vi "Set Parameters File MD5 Checksum.vi"(8 "error in":errorcluster, 9 "MD5":string, 11 "custom device ref":T1 format="%.0x") -> (0 "error out":errorcluster, 3 "custom device ref out":T1 format="%.0x")   [LabVIEW 2024, in "AIM ARINC 429 Scripting.lvlib"]
uses:
  AIM ARINC 429 Scripting.lvlib
  <vilib>/NI VeriStand/Custom Device API/Custom Device Item Ref.ctl
  Constants.vi
  <vilib>/NI VeriStand/Custom Device API/Set Item Property (String).vi
  <vilib>/NI VeriStand/Custom Device API/Custom Device API.lvlib
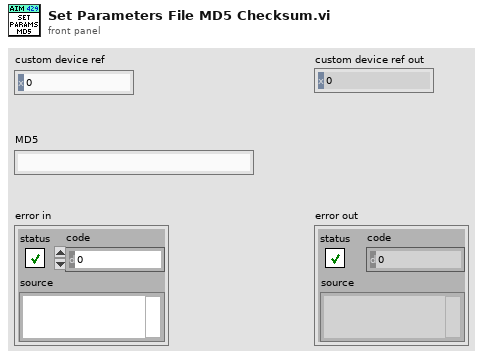
[diagram p1: front panel]
types:
  T1 = typedef "Custom Device API.lvlib/Custom Device Item Ref.ctl" = u64
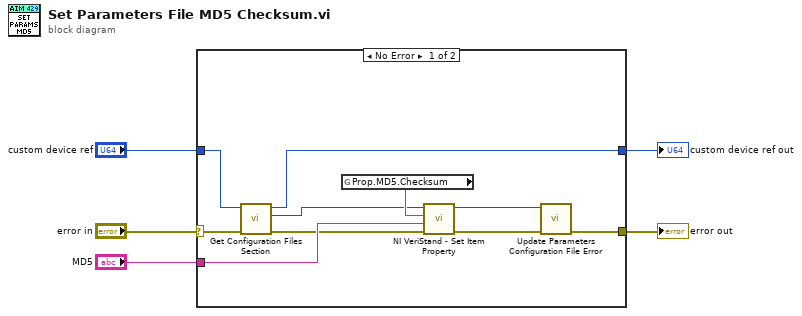
[diagram p0: block diagram]
diagram:
  n1 = case shown="No Error" "error in" {
    selector: "error in" -> [w10 w17]
    tunnel: "custom device ref" -> [w7 w16]
    tunnel: [w11 w17] -> w4
    tunnel: "MD5" -> [w15 _]
    tunnel: [w6 w16] -> w1
    frame No Error {
      n2 = call "Get Configuration Files Section.vi"("error in"=w10, "custom device ref"=w7) -> ("error out"=w9:errorcluster, "configuration files ref"=w8:T1, "custom device ref out"=w6:T1)  [unwired: 7 in]
      n3 = global read "Constants.vi" "Prop.MD5.Checksum"() -> (w14:string)
      n4 = call-poly <vilib>:"NI VeriStand - Set Item Property.vi"("error in (no error)"=w9, "Value"=w15, "Property Name"=w14, "Item Ref in"=w8) -> ("error out"=w12:errorcluster, "Item Ref out"=w13:T1)  [unwired: 5 in, 1 out]
      n5 = call "Update Parameters Configuration File Error.vi"("error in"=w12, "configuration files ref"=w13) -> ("error out"=w11:errorcluster)  [unwired: 8 in, 1 out]
    }
    frame Error {
    }
  }
  "error out" <- w4
  "custom device ref out" <- w1
